vi "stateMachine_dualVStim.vi"() -> ()   [LabVIEW 2014]
uses:
  daq_channel_read_parameter.ctl
  <vilib>/Platform/TimedLoop/XDataNode/timing_clust.ctl
  <vilib>/Platform/TimedLoop/XDataNode/nitl_modes.ctl
  <vilib>/Platform/TimedLoop/XDataNode/wakeup.ctl
  <vilib>/dex/Stream Element Allocation Mode.ctl
  states_def.ctl
  UDP_Para_def.ctl
  <vilib>/DAQmx/write.llb/DAQmx Write (Digital 1D Bool NChan 1Samp 1Line).vi
  <vilib>/platform/TimedLoop/XDataNode/XDataNode.xnode
  <vilib>/Platform/TimedLoop/XDataNode/XDNodeRunTimeDep.lvlib
  <resource>/objmgr/ni.dex.rc
panel:
  out "rightcounter":i32
  out "leftcounter":i32
  out "beh type":string
  out "vs type":string
  out "Tab Control":enum32{"State Machine"}(tab)
  in  "vsFilterPeriod_uS":i32=500 format="%#1.6f"
  in  "lickThreshold_V":fxp<+/-,16,5> format="%#.4g"
  in  "vsThreshold_V":fxp<+/-,16,5> format="%#.4g"
  in  "audioThreshold_V":fxp<+/-,16,5> format="%#.4g"
  in  "audioFilterPeriod_uS":i32=50000 format="%#1.6f"
  in  "audioOffState_V":fxp<+/-,16,5> format="%#.4g"
  out "rtFIFOsize":u32=50
  out "rtFIFOtimeout":u32
  out "rtFIFOdataPool":u32=50
  out "stateMachineCycle_uS":i64=500
  out "(Actual)":i64
  in  "delay_uS":u32
  out "IP_RT":string="192.168.137.2"
  in  "port_broadcast":u16=9091
  out "IP_host":string="192.168.137.1"
  out "port_host":u16=9090
  in  "Tab Control 2":enum32{"Data Transfer"}(tab)
  out "stream counter":u32
  out "Is Connected":bool
  out "Available Elements for Writing":i32
  out "stream writer buffer size":i32=500
  in  "rewardPeriod_uS":u32
  in  "waterOn_uS":u32
  in  "timeout_uS":u32=5000000
  in  "shockOn_uS":u32
  in  "Stop state":bool
  out "Initial data received":bool
  out "Tab Control 3":enum32{"Current status"}(tab)
  in  "toneReward":bool
  out "ABORT":bool
  out "trialStart":bool
  out "trialDone":bool
  out "Busy":bool
  out "stateLatched":bool
  out "curKey":u32=1
  out "curState":u32
  out "rtFIFOdataDim":i32
  in  "actuatorOn":bool
  in  "manualWaterRight":bool
  in  "manualWaterLeft":bool
  in  "lickReward":bool
  in  "allowPunish":bool
  in  "forceLRswitch":bool
  in  "allowCorrection":bool
  in  "allowAutoWater":bool
  out "error out":errorcluster
  in  "trialKey":i32[](array[numeric])
  in  "rwdrefPeriod_uS":u32
  out "FlagWaterLeft":bool
  in  "chanellParaCluster":T1={"audioOffState_V"=0.0, "audioFilterPeriod_uS"=50000, "audioThreshold_V"=0.0, "vsThreshold_V"=0.0, "vsFilterPeriod_uS"=0, "lickThreshold_V"=0.0} {"vsFilterPeriod_uS" format="%#1.6f"; "audioFilterPeriod_uS" format="%#1.6f"}
  out "leftWaterOnFlag":bool
  out "rightWaterOnFlag":bool
  out "contNoReward":i32
  out "rewardStatus":bool
  in  "timeVS_uS":u32=2000000
  in  "timeTravel_uS":i32=400000
  out "skipRewFlag":bool
types:
  T1 = typedef "daq_channel_read_parameter.ctl" = cluster{"audioOffState_V":fxp<+/-,16,5>, "audioFilterPeriod_uS":i32, "audioThreshold_V":fxp<+/-,16,5>, "vsThreshold_V":fxp<+/-,16,5>, "vsFilterPeriod_uS":i32, "lickThreshold_V":fxp<+/-,16,5>}
  T2 = typedef "XDNodeRunTimeDep.lvlib/timing_clust.ctl" = cluster{"Expected End [f-1]":u64, "Actual End [f-1]":u64, "Finished Late? [f-1]":bool, "Expected End [i-1]":u64, "Actual End [i-1]":u64, "Finished Late? [i-1]":bool, "Expected Start [i]":u64, "Actual Start [i]":u64, "Expected Start [f]":u64, "Actual Start [f]":u64, "Source Name":string, "Structure Name":string, "Period":i64, "Deadline":i64, "Offset":i64, "Start":i64, "Priority":i32, "Timeout":i32, "Mode":T3, "Wakeup Reason":T4, "Error":errorcluster, "Source Type":string, "Secondary Source Type":string, "Global End Time":u64, "Global Start Time":u64, "Frame Duration":u64, "Iteration Duration":u64, "Assigned CPU":i32, "I/O Scan Engine Mode":u32}
  T3 = typedef "XDNodeRunTimeDep.lvlib/nitl_modes.ctl" = enum32{"No Change", "Process missed periods, maintain original phase", "Discard missed periods, maintain original phase", "Process missed periods, ignore original phase", "Discard missed periods, ignore original phase"}
  T4 = typedef "XDNodeRunTimeDep.lvlib/wakeup.ctl" = enum32{"Normal", "Aborted", "Asynchronous wakeup", "Timing source error", "Timed loop error", "Timeout"}
  T5 = typedef "states_def.ctl" = enum16{"idle", "vs before", "vs", "vs after", "delay", "tone before", "tone", "tone after", "cycle end", "reward", "reward refractory", "punish", "punish refractory", "timeout", "exit", "manualwater"}
  T6 = typedef "Stream Element Allocation Mode.ctl" = u32
  T7 = typedef "UDP_Para_def.ctl" = enum16{"no", "start", "stop", "dly", "rwp", "rwf", "wdr", "shd", "tod", "lkr", "tlr", "alp", "msh", "mwl", "mwr", "alc", "lth", "vth", "ath", "aof", "afp", "vfp"}
  T8 = cluster{"leftLick":bool, "rightLick":bool, "visualStimuli2":bool, "tone":bool, "visualStimuli1":bool}
  T9 = cluster{"leftLick":dbl, "rightLick":dbl, "visualStimuli2":dbl, "tone":dbl, "visualStimuli1":dbl}
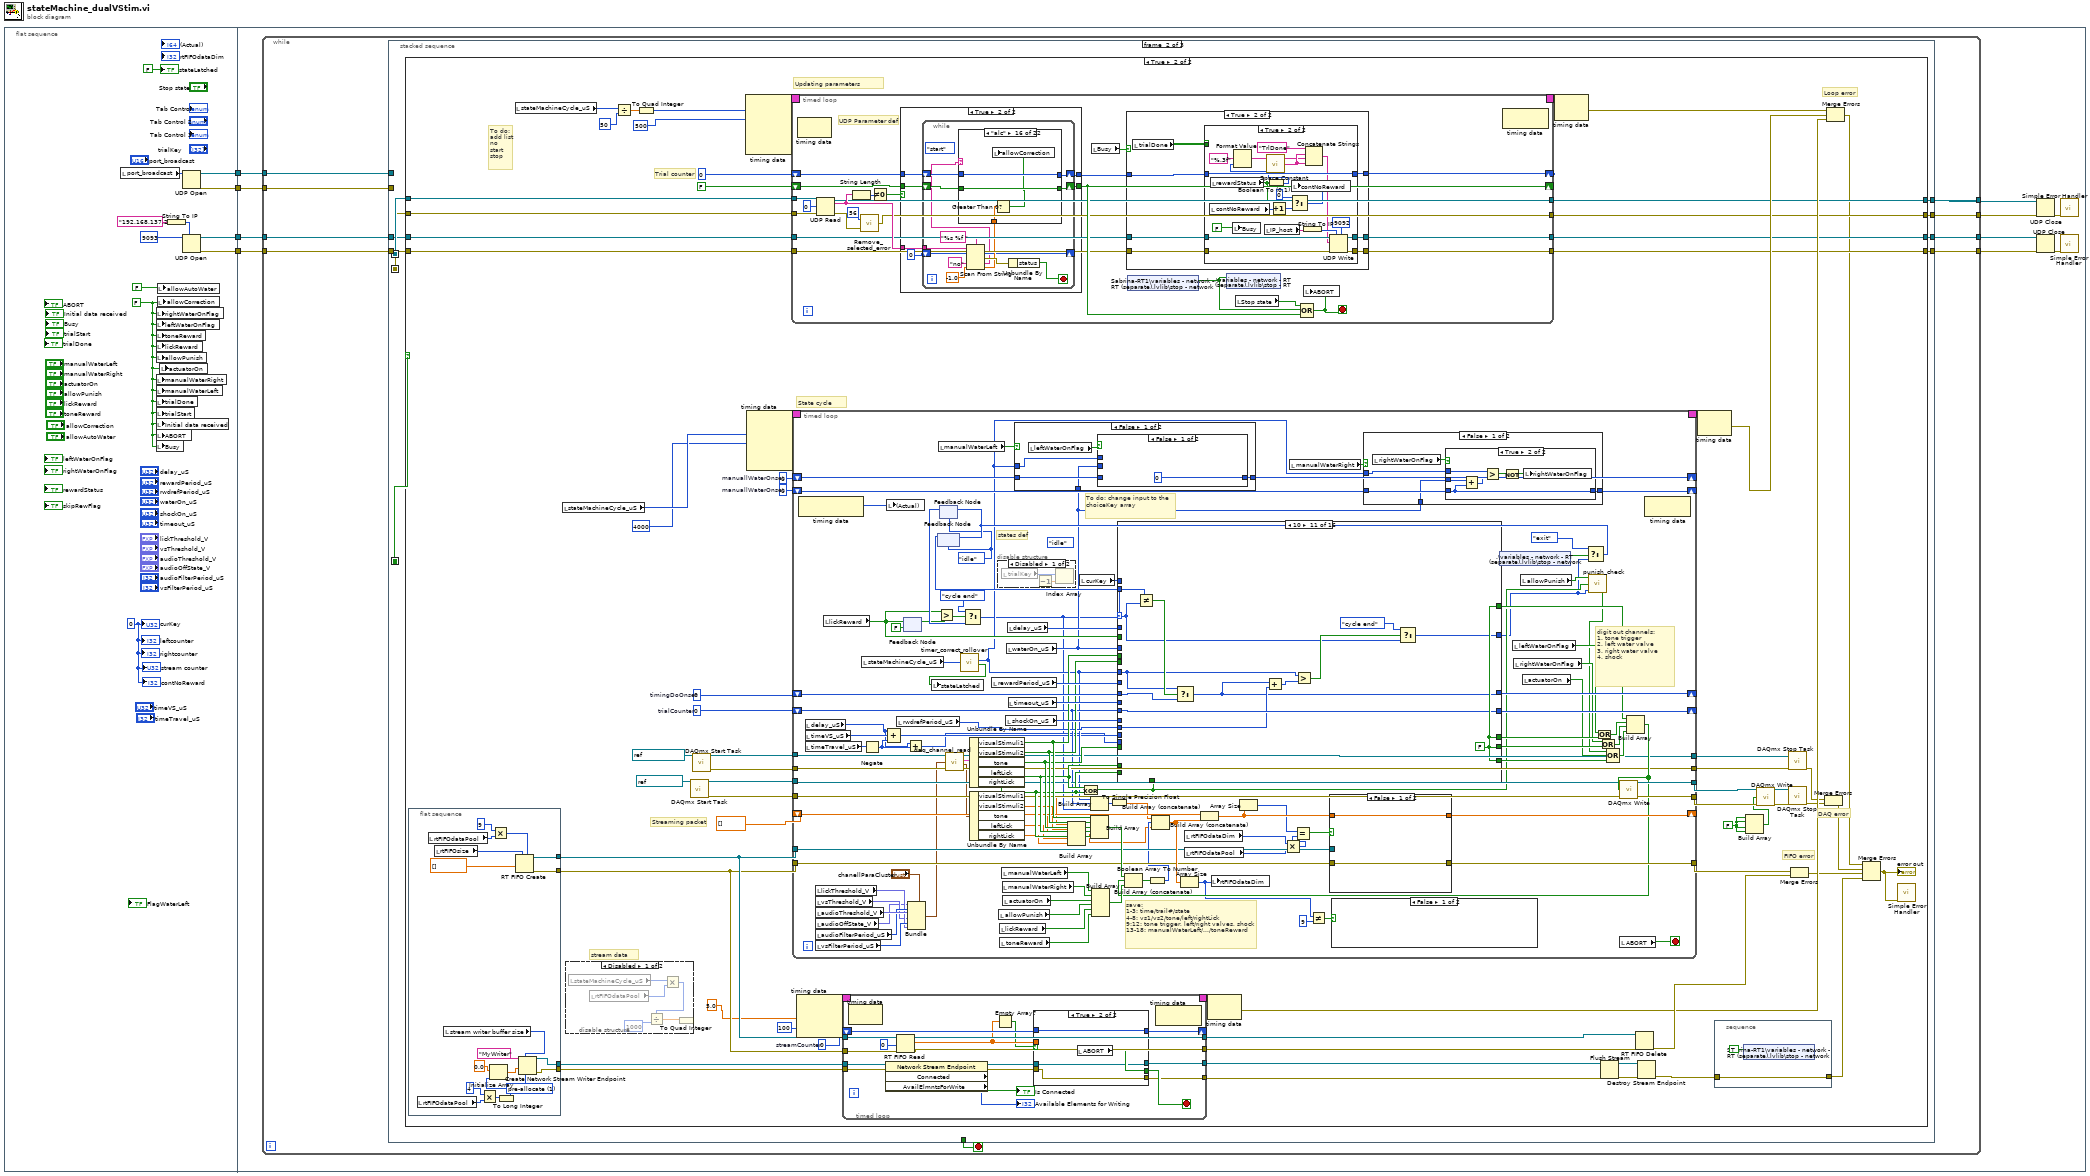
[diagram p0: block diagram]
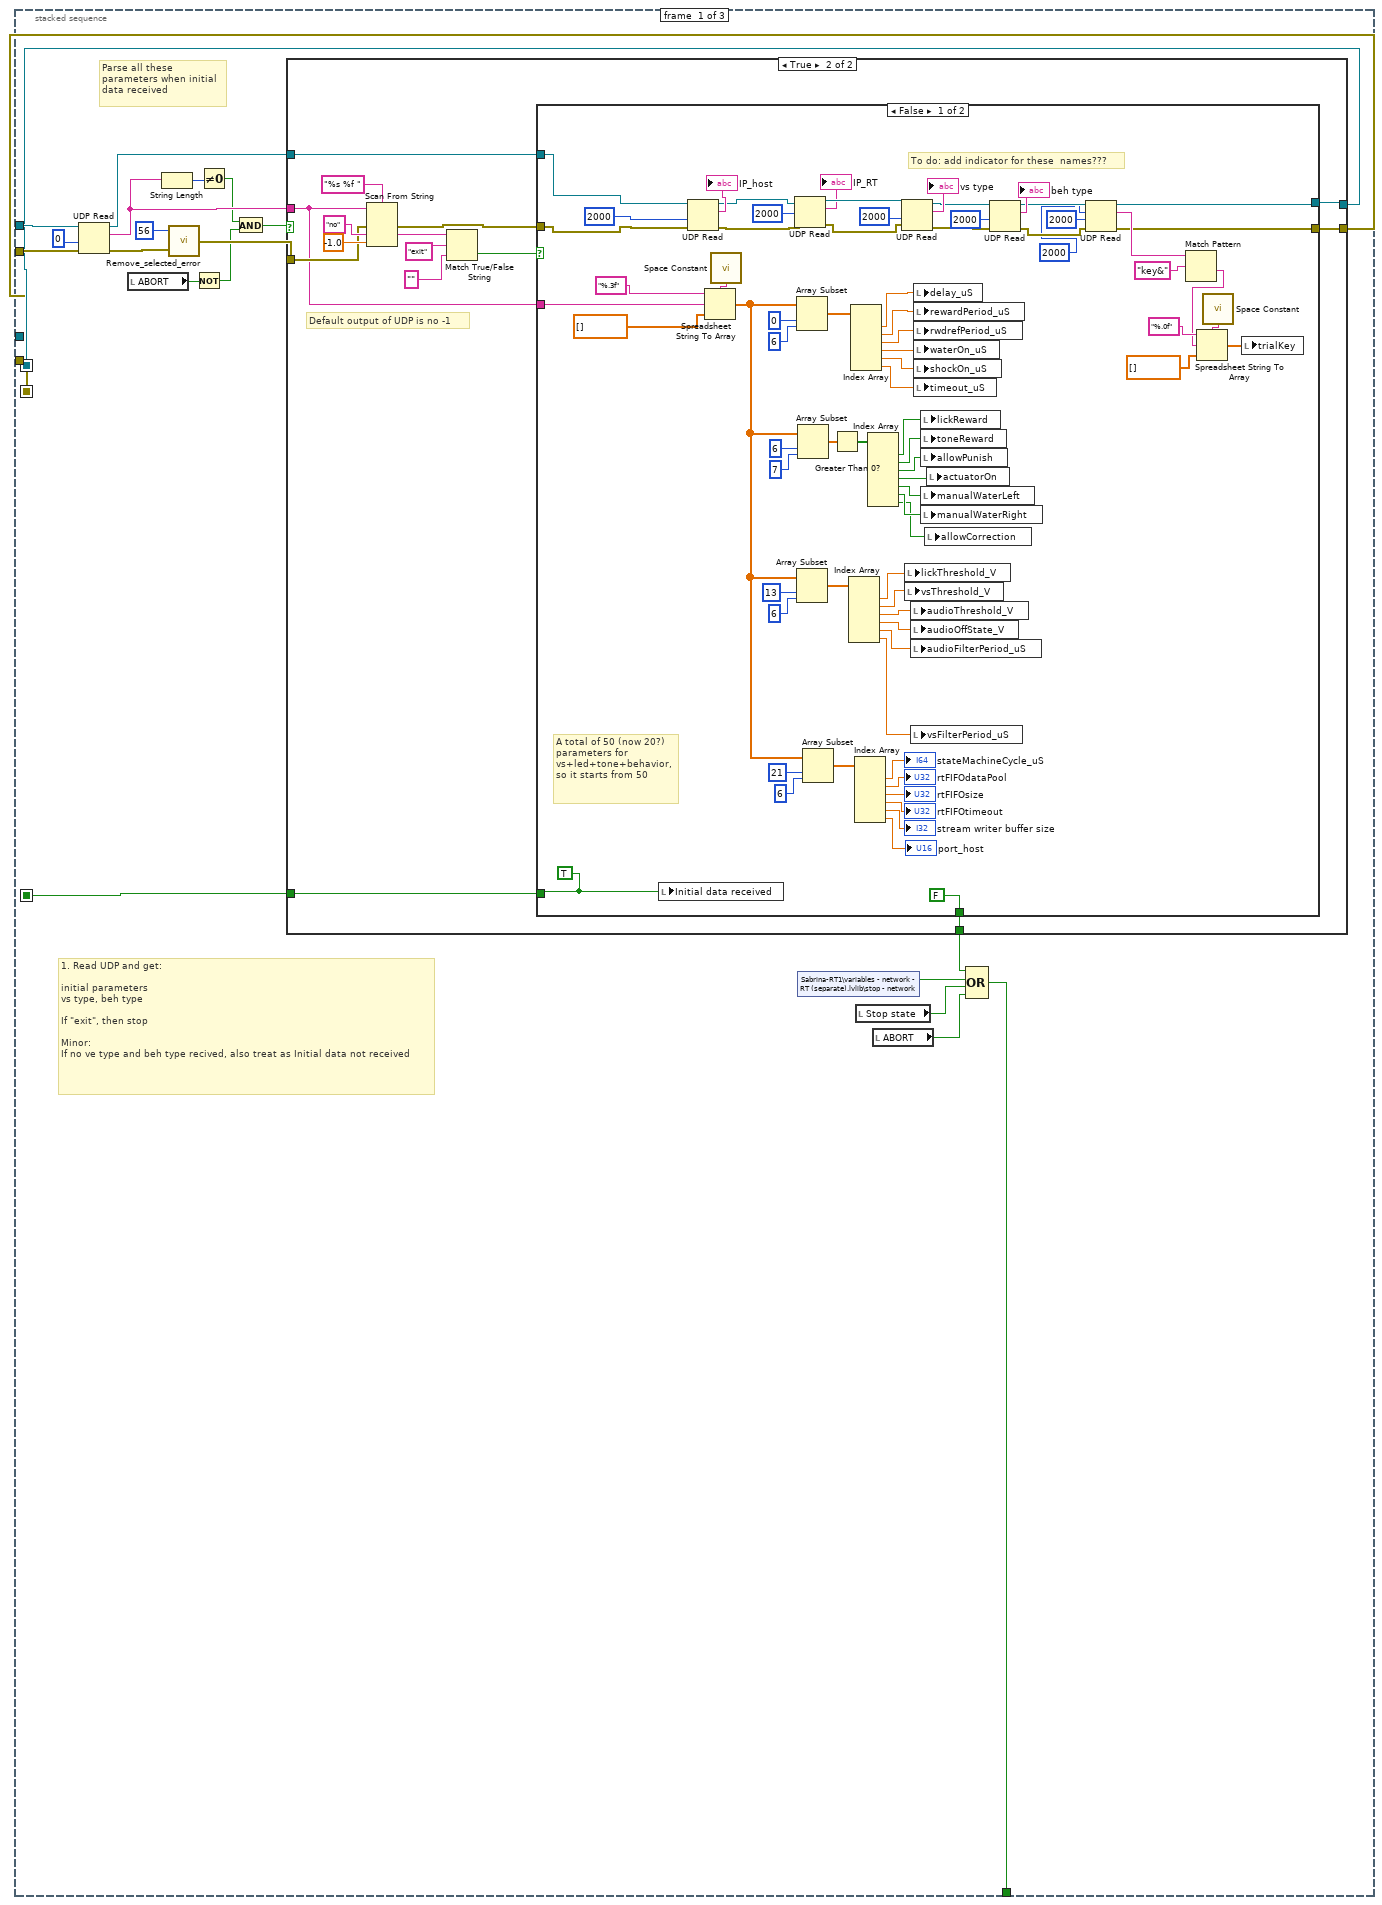
[diagram p2: hidden frame]
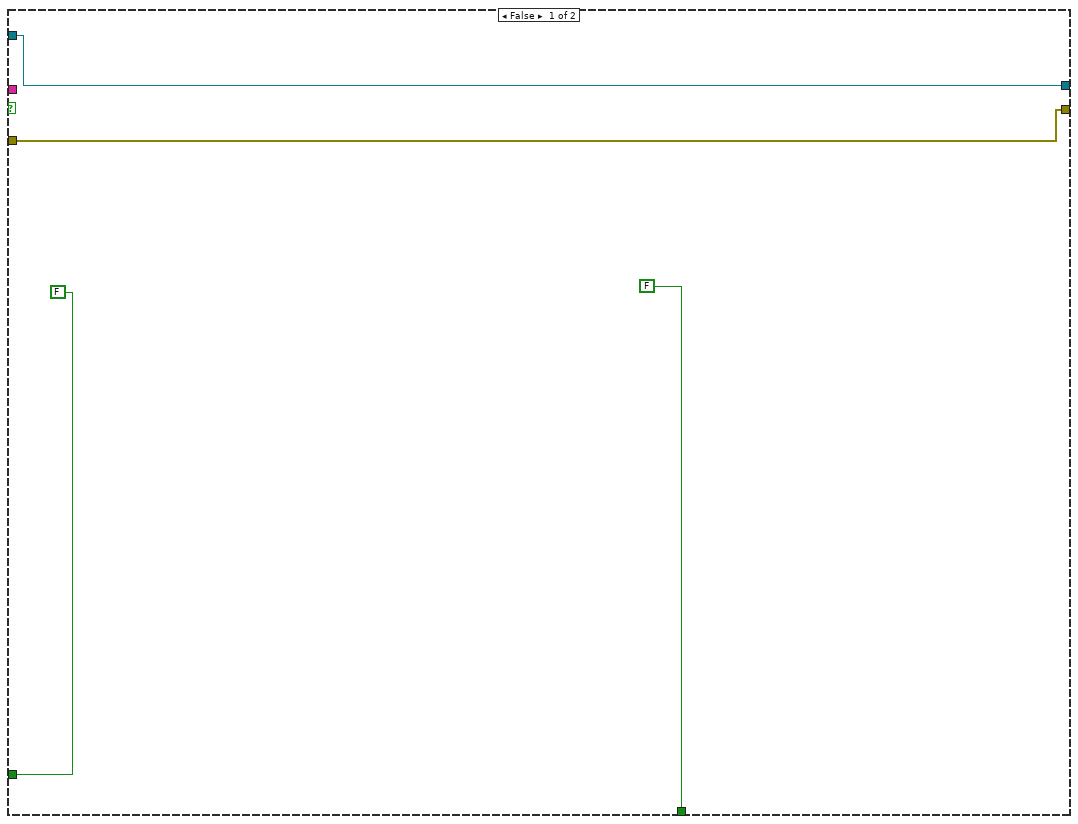
[diagram p3: hidden frame]
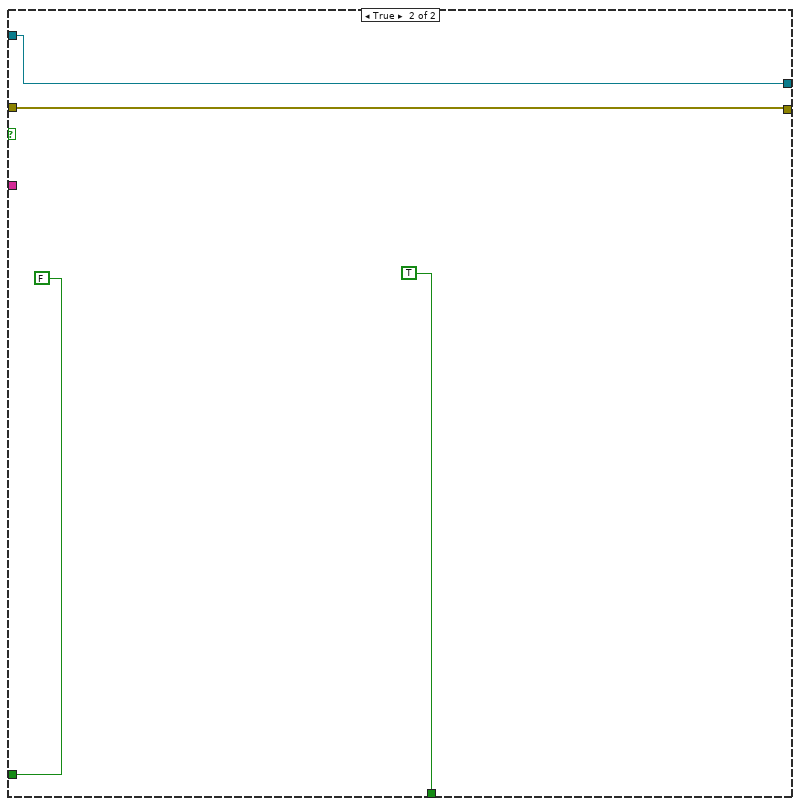
[diagram p4: hidden frame]
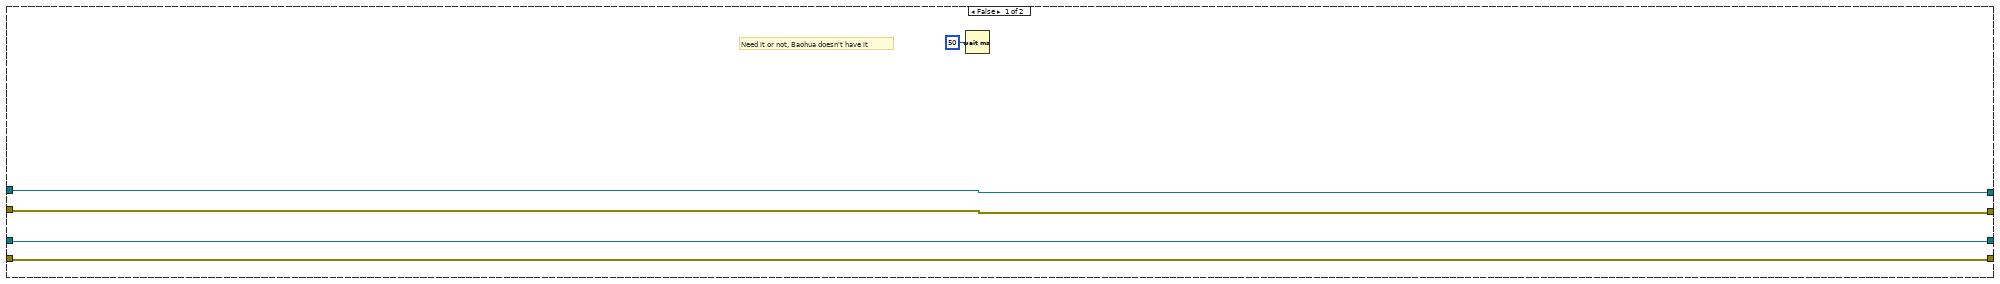
[diagram p5: hidden frame]
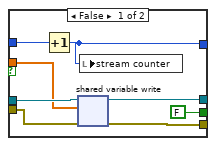
[diagram p7: hidden frame]
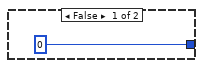
[diagram p9: hidden frame]
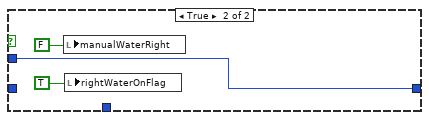
[diagram p10: hidden frame]
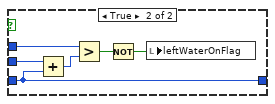
[diagram p11: hidden frame]
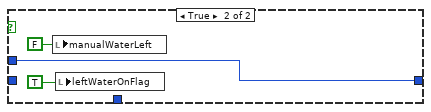
[diagram p12: hidden frame]
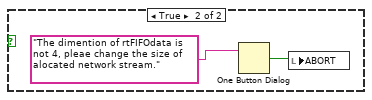
[diagram p13: hidden frame]
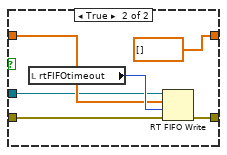
[diagram p14: hidden frame]
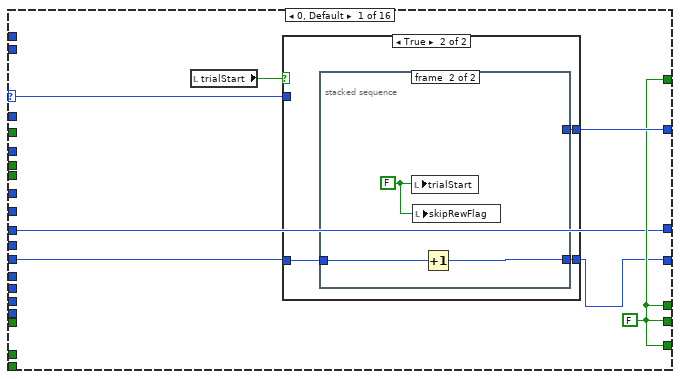
[diagram p15: hidden frame]
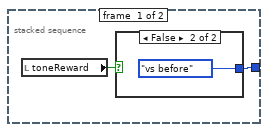
[diagram p17: hidden frame]
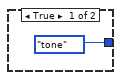
[diagram p18: hidden frame]
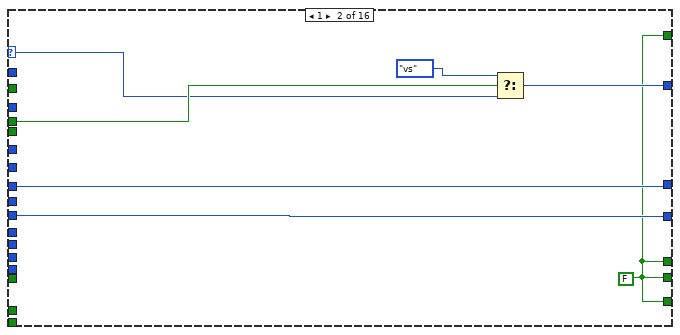
[diagram p19: hidden frame]
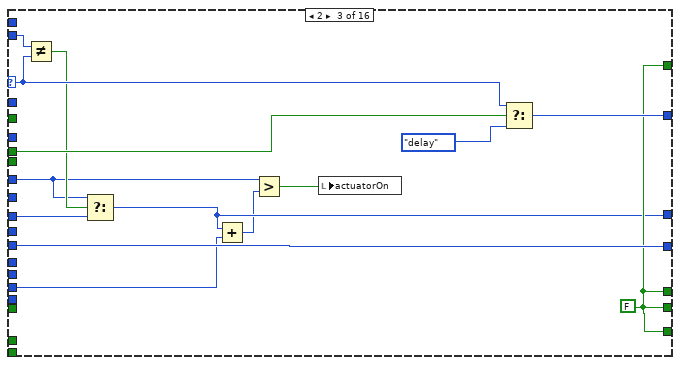
[diagram p20: hidden frame]
diagram:
  n1 = flat-sequence {
    tunnel: [w16] -> w4
    tunnel: [w15] -> w3
    tunnel: [w11] -> w2
    tunnel: [w10] -> w1
    tunnel: w4 -> [w26]
    tunnel: w3 -> [w25]
    tunnel: w2 -> [w21]
    tunnel: w1 -> [w20]
    frame #0 {
      w7 = FALSE
      w6 = 0
      n2 = local read "port_broadcast"() -> (w14:u16)
      n3 = local write "rightWaterOnFlag"(w7) -> ()
      n4 = local write "leftWaterOnFlag"(w7) -> ()
      n5 = local write "toneReward"(w7) -> ()
      n6 = local write "lickReward"(w7) -> ()
      n7 = local write "allowPunish"(w7) -> ()
      n8 = local write "manualWaterRight"(w7) -> ()
      n9 = local write "manualWaterLeft"(w7) -> ()
      n10 = local write "trialDone"(w7) -> ()
      n11 = local write "trialStart"(w7) -> ()
      n12 = local write "Initial data received"(w7) -> ()
      n13 = local write "ABORT"(w7) -> ()
      n14 = local write "Busy"(w7) -> ()
      n15 = local write "allowAutoWater"(FALSE) -> ()
      n16 = local write "allowCorrection"(w7) -> ()
      n17 = local write "actuatorOn"(w7) -> ()
      n18 = String To IP(1:"192.168.137.2") -> (0:w8:u32)
      n19 = UDP Open(7:w8, 11:u16 9093) -> (port=w11:refnum<k16>, 0:w10:errorcluster)  [unwired: 3 in, 1 out]
      n20 = UDP Open(11:w14) -> (port=w16:refnum<k16>, 0:w15:errorcluster)  [unwired: 4 in, 1 out]
      "stateLatched" <- FALSE
      "curKey" <- w6
      "leftcounter" <- w6
      "rightcounter" <- w6
      "stream counter" <- w6
      "contNoReward" <- w6
    }
    frame #1 {
      n21 = while {
        tunnel: w26 -> [w35]
        tunnel: w25 -> [w34]
        tunnel: [w32] -> w23
        tunnel: [w31] -> w22
        tunnel: w21 -> [w30]
        tunnel: w20 -> [w29]
        tunnel: [w28] -> w19
        tunnel: [w27] -> w18
        stop <- w33 stop-if-true
        n22 = stacked-sequence {
          seq-local: [w45 _ _] -> [_ w162 _]
          seq-local: [w37 _ _] -> [_ w159 _]
          seq-local: [w36 _ _] -> [_ w158 _]
          tunnel: w35 -> [w56 _ _]
          tunnel: w34 -> [w55 _ _]
          tunnel: [w46 _ _] -> w33
          tunnel: [_ w161 _] -> w32
          tunnel: [_ w160 _] -> w31
          tunnel: w30 -> [_ w157 _]
          tunnel: w29 -> [_ w154 _]
          tunnel: [_ w156 _] -> w28
          tunnel: [_ w155 _] -> w27
          frame #0 {
            # "Parse all these \nparameters when initial\ndata received"
            # "1. Read UDP and get:\n\ninitial parameters\nvs type, beh type\n\nIf \"exit\", then stop\n\nMinor:\nIf no ve type and beh type recived, also treat as Initial data not received"
            n23 = UDP Read(connection ID=w56, timeout ms (25000)=0, 8:w55) -> (data out=w53:string, error out=w43:errorcluster, 3:w54:refnum<k16>)  [unwired: 1 in, 2 out]
            n24 = local read "ABORT"() -> (w41:bool)
            n25 = String Length(string=w53) -> (length=w52:i32)
            n26 = call "Remove_selected_error.vi"("error in (no error)"=w43, "errorCode"=56 ("timeout ms (25000)")) -> ("error out"=w44:errorcluster)
            n27 = Not(x=w41) -> (.not. x?=w38:bool)
            n28 = Not Equal To 0?(x=w52) -> (x != 0?=w39:bool)
            n29 = And(x=w39, y=w38) -> (x .and. y?=w40:bool)
            n30 = case shown="True" w40 {
              tunnel: w53 -> [_ w65]
              tunnel: w54 -> [w58 w66]
              tunnel: w44 -> [w57 w73]
              tunnel: [FALSE w64] -> w50
              tunnel: [FALSE w63] -> w45
              tunnel: [w58 w62] -> w37
              tunnel: [w57 w61] -> w36
              frame False {
              }
              frame True {
                # "Default output of UDP is no -1"
                n31 = Scan From String(format string="%s %f ", input string=w65, error in=w73, default 1="no" ("default value 1"), default 2=sgl -1.0 ("default value 1")) -> (error out=w67:errorcluster, output 1=w72:string)  [unwired: 2 in, 2 out]
                n32 = Match True/False String(2:"" ("false string"), 3:"exit" ("true string"), 4:w72) -> (0:w68:bool)  [unwired: 1 out]
                n33 = case shown="False" w68 {
                  tunnel: w67 -> [w111 w151]
                  tunnel: w66 -> [w112 w150]
                  tunnel: w65 -> [w143 _]
                  tunnel: [FALSE TRUE] -> w64
                  tunnel: [w141 FALSE] -> w63
                  tunnel: [w78 w150] -> w62
                  tunnel: [w77 w151] -> w61
                  frame False {
                    w141 = TRUE
                    # "A total of 50 (now 20?) parameters for vs+led+tone+behavior, so it starts from 50"
                    # "To do: add indicator for these  names???"
                    n34 = local write "Initial data received"(w141) -> ()
                    n35 = UDP Read(connection ID=w112, timeout ms (25000)=2000, 8:w111) -> (data out=→"IP_host":string, error out=w110:errorcluster, 3:w108:refnum<k16>)  [unwired: 1 in, 2 out]
                    n36 = call <vilib>:"Space Constant.vi"() -> ("String"=w148:string)
                    n37 = Spreadsheet String To Array(delimiter (Tab)=w148, format string="%.3f", spreadsheet string=w143, array type (2D Dbl)=sgl[] []) -> (array=w119:sgl[])
                    n38 = UDP Read(connection ID=w108, timeout ms (25000)=2000, 8:w110) -> (data out=→"IP_RT":string, error out=w109:errorcluster, 3:w107:refnum<k16>)  [unwired: 1 in, 2 out]
                    n39 = Array Subset(array=w119, index=0 ("timeout ms (25000)"), length=6 ("timeout ms (25000)")) -> (w137:sgl[])
                    n40 = Array Subset(array=w119, index=13 ("timeout ms (25000)"), length=6 ("timeout ms (25000)")) -> (w133:sgl[])
                    n41 = Array Subset(array=w119, index=6 ("timeout ms (25000)"), length=7 ("timeout ms (25000)")) -> (w130:sgl[])
                    n42 = Array Subset(array=w119, index=21 ("timeout ms (25000)"), length=6 ("timeout ms (25000)")) -> (w120:sgl[])
                    n43 = Greater Than 0?(x=w130) -> (x > 0?=w129:bool[])
                    n44 = Index Array(array=w133) -> (element #1=w95:sgl, element #2=w94:sgl, element #3=w93:sgl, element #4=w92:sgl, element #5=w91:sgl, element #6=w90:sgl)  [unwired: 6 in]
                    n45 = Index Array(array=w137) -> (element #1=w101:sgl, element #2=w100:sgl, element #3=w99:sgl, element #4=w98:sgl, element #5=w97:sgl, element #6=w96:sgl)  [unwired: 6 in]
                    n46 = Index Array(array=w120) -> (element #1=→"stateMachineCycle_uS":sgl, element #2=→"rtFIFOdataPool":sgl, element #3=→"rtFIFOsize":sgl, element #4=→"rtFIFOtimeout":sgl, element #5=→"stream writer buffer size":sgl, element #6=→"port_host":sgl)  [unwired: 6 in]
                    n47 = Index Array(array=w129) -> (element #1=w128:bool, element #2=w127:bool, element #3=w126:bool, element #4=w125:bool, element #5=w124:bool, element #6=w123:bool, element #7=w76:bool)  [unwired: 7 in]
                    n48 = UDP Read(connection ID=w107, timeout ms (25000)=2000, 8:w109) -> (data out=→"vs type":string, error out=w140:errorcluster, 3:w139:refnum<k16>)  [unwired: 1 in, 2 out]
                    n49 = local write "lickThreshold_V"(w95) -> ()
                    n50 = local write "vsThreshold_V"(w94) -> ()
                    n51 = local write "audioThreshold_V"(w93) -> ()
                    n52 = local write "audioOffState_V"(w92) -> ()
                    n53 = local write "audioFilterPeriod_uS"(w91) -> ()
                    n54 = local write "vsFilterPeriod_uS"(w90) -> ()
                    n55 = local write "delay_uS"(w101) -> ()
                    n56 = local write "rewardPeriod_uS"(w100) -> ()
                    n57 = local write "rwdrefPeriod_uS"(w99) -> ()
                    n58 = local write "waterOn_uS"(w98) -> ()
                    n59 = local write "shockOn_uS"(w97) -> ()
                    n60 = local write "timeout_uS"(w96) -> ()
                    n61 = local write "lickReward"(w128) -> ()
                    n62 = local write "toneReward"(w127) -> ()
                    n63 = local write "allowPunish"(w126) -> ()
                    n64 = local write "manualWaterLeft"(w124) -> ()
                    n65 = local write "manualWaterRight"(w123) -> ()
                    n66 = local write "allowCorrection"(w76) -> ()
                    n67 = local write "actuatorOn"(w125) -> ()
                    n68 = UDP Read(connection ID=w139, timeout ms (25000)=2000, 8:w140) -> (data out=→"beh type":string, error out=w87:errorcluster, 3:w88:refnum<k16>)  [unwired: 1 in, 2 out]
                    n69 = UDP Read(connection ID=w88, max size (548)=2000 ("timeout ms (25000)"), timeout ms (25000)=2000, 8:w87) -> (data out=w82:string, error out=w77:errorcluster, 3:w78:refnum<k16>)  [unwired: 2 out]
                    n70 = Match Pattern(string=w82, regular expression="key&") -> (after substring=w80:string)  [unwired: 1 in, 3 out]
                    n71 = call <vilib>:"Space Constant.vi"() -> ("String"=w85:string)
                    n72 = Spreadsheet String To Array(delimiter (Tab)=w85, format string="%.0f", spreadsheet string=w80, array type (2D Dbl)=dbl[] []) -> (array=w83:dbl[])
                    n73 = local write "trialKey"(w83) -> ()
                  }
                  frame True {
                  }
                }
              }
            }
            n74 = shared-variable "Sabrina-RT1\\variables - network - RT (separate).lvlib\\stop - network"() -> (w49:bool)  [unwired: 1 in, 1 out]
            n75 = local read "Stop state"() -> (w48:bool)
            n76 = local read "ABORT"() -> (w47:bool)
            n77 = Compound Arithmetic op=OR(w50, w49, w48, w47) -> (w46:bool)
          }
          frame #1 {
            n78 = case shown="True" w162 {
              tunnel: w159 -> [w166 w212]
              tunnel: w158 -> [w165 w211]
              tunnel: [w166 w184] -> w161
              tunnel: [w165 w185] -> w160
              tunnel: w157 -> [w164 w189]
              tunnel: w154 -> [w163 w188]
              tunnel: [w163 w187] -> w156
              tunnel: [w164 w186] -> w155
              frame False {
                # "Need it or not, Baohua doesn't have it"
                n79 = Wait (ms)(milliseconds to wait=u32 50) -> ()  [unwired: 1 out]
              }
              frame True {
                w168 = 0  # manuallWaterOnset
                w169 = 0  # manuallWaterOnset
                w195 = FALSE
                w224 = 0  # streamCounter
                w227 = 0  # timingDoOnset
                w226 = 0  # trialCounter
                # "Streaming packet"
                # "Trial counter"
                # "Loop error"
                # "DAQ error"
                # "FIFO error"
                # "Updating parameters"
                # "State cycle"
                # "To do:\nadd list\nno\nstart\nstop"
                # "stream data"
                n80 = flat-sequence {
                  tunnel: [w254] -> w229
                  tunnel: [w253] -> w228
                  tunnel: [w252] -> w215
                  tunnel: [w251] -> w214
                  frame #0 {
                    w258 = T6 1 items=["allocate as needed", "pre-allocate"] ("element allocation mode")
                    n81 = local read "rtFIFOdataPool"() -> (w249:u32)
                    n82 = local read "rtFIFOdataPool"() -> (w246:u32)
                    n83 = local read "rtFIFOsize"() -> (w260:u32)
                    n84 = local read "stream writer buffer size"() -> (w250:i32)
                    n85 = Multiply(x=u32 4, y=w249) -> (x*y=w244:u32)
                    n86 = Multiply(x=9, y=w246) -> (x*y=w245:u32)
                    n87 = To Long Integer(number=w244) -> (32bit integer=w243:i32)
                    n88 = Initialize Array(sgl 0.0, w243) -> (w257:sgl[])
                    n89 = RT FIFO Create(1:sgl[] [], 4:w260, 6:w245) -> (8:w252:refnum<k33>, 11:w251:errorcluster)  [unwired: 5 in, 1 out]
                    n90 = Create Network Stream Writer Endpoint(6:w258, 7:w250, 9:w257, 11:"MyWriter" ("writer name")) -> (0:w254:errorcluster, 3:w253:refnum<k21>)  [unwired: 3 in]
                  }
                }
                n91 = local read "stateMachineCycle_uS"() -> (w213:i64)
                n92 = local read "stateMachineCycle_uS"() -> (w223:i64)
                n93 = disable-structure shown="Disabled" {
                  frame Disabled {
                    n94 = local read "stateMachineCycle_uS"() -> (w238:i64)
                    n95 = local read "rtFIFOdataPool"() -> (w237:u32)
                    n96 = Multiply(x=w238, y=w237) -> (x*y=w239:i64)
                    n97 = Divide(x=w239, y=i64 1000) -> (x/y=w236:dbl)
                    n98 = To Quad Integer(1:w236) -> ()  [unwired: 1 out]
                  }
                  frame Enabled {
                  }
                }
                n99 = Divide(x=w213, y=i64 50) -> (x/y=w219:dbl)
                n100 = To Quad Integer(1:w219) -> (0:w218:i64)
                n101 = call <vilib>:"DAQmx Start Task.vi"("task/channels in"=refnum<k21> "digitWrite" ("digitWrite")) -> ("task out"=w181:refnum<k21>, "error out"=w180:errorcluster)  [unwired: 13 in]
                n102 = call <vilib>:"DAQmx Start Task.vi"("task/channels in"=refnum<k21> "analogRead" ("DAQmx Task Name")) -> ("task out"=w171:refnum<k21>, "error out"=w170:errorcluster)  [unwired: 13 in]
                n103 = node-c288(w218, 500 ("Priority")) -> (w235:T2)  [unwired: 3 in]
                n104 = node-c288(w223, 4000 ("Priority")) -> (w233:T2)  [unwired: 3 in]
                n105 = timed-loop {
                  timing: w235 -> [_]
                  timing-out: [_] -> w234
                  shift-right: [w761] -> _
                  shift-left: 0 ("timeout ms (25000)") -> [w763]
                  shift-right: [w757] -> _
                  shift-left: FALSE -> [w760]
                  tunnel: [w754] -> w186
                  tunnel: [w753] -> w187
                  tunnel: w212 -> [w752]
                  tunnel: w211 -> [w751]
                  tunnel: w189 -> [w745]
                  tunnel: w188 -> [w748]
                  tunnel: [w747] -> w185
                  tunnel: [w746] -> w184
                  stop <- w759 stop-if-true
                  # "UDP Parameter def"
                  n106 = node-c288() -> ()  [unwired: 1 in, 1 out]
                  n107 = UDP Read(connection ID=w752, timeout ms (25000)=0, 8:w751) -> (data out=w764:string, error out=w750:errorcluster, 3:w746:refnum<k16>)  [unwired: 1 in, 2 out]
                  n108 = String Length(string=w764) -> (length=w766:i32)
                  n109 = call "Remove_selected_error.vi"("error in (no error)"=w750, "errorCode"=56 ("timeout ms (25000)")) -> ("error out"=w747:errorcluster)
                  n110 = Not Equal To 0?(x=w766) -> (x != 0?=w765:bool)
                  n111 = case shown="True" w765 {
                    tunnel: w764 -> [_ w808]
                    tunnel: w763 -> [w802 w807]
                    tunnel: [w802 w806] -> w762
                    tunnel: w760 -> [w801 w805]
                    tunnel: [w801 w804] -> w757
                    frame False {
                    }
                    frame True {
                      n112 = while {
                        tunnel: w808 -> [w822]
                        shift-right: [w810] -> _
                        shift-left: 0 ("timeout ms (25000)") -> [w811]
                        shift-right: [w815] -> w806
                        shift-left: w807 -> [w816]
                        shift-right: [w813] -> w804
                        shift-left: w805 -> [w814]
                        stop <- w817 stop-if-true
                        (unwired) UDP_Para_def."start"
                        n113 = Scan From String(format string="%s %f ", input string=w822, initial scan location=w811, default 1="no" ("default value 1"), default 2=-1.0 ("default value 2")) -> (offset past scan=w810:u32, error out=w818:errorcluster, output 1=w809:string, output 2=w812:dbl)  [unwired: 1 in, 1 out]
                        n114 = case shown="\"alc\"" w809 {
                          tunnel: [w824 w826 w835 w837 w842 w847 w852 w857 w862 w867 w871 w875 w879 w883 w887 w892 w895 w899 w903 w907 w911 w916] -> w815
                          tunnel: w816 -> [w824 w827 w835 w837 w842 w847 w852 w857 w862 w867 w871 w875 w879 w883 w887 w892 w895 w899 w903 w907 w911 w916]
                          tunnel: [w823 w831 w832 w836 w841 w846 w851 w856 w861 w866 w870 w874 w878 w882 w886 w891 w894 w898 w902 w906 w910 w915] -> w813
                          tunnel: w814 -> [w823 w831 w833 w836 w841 w846 w851 w856 w861 w866 w870 w874 w878 w882 w886 w891 w894 w898 w902 w906 w910 w915]
                          tunnel: w812 -> [_ w828 _ w839 w844 w849 w854 w859 w864 w869 w873 w877 w881 w885 w889 w893 w897 w901 w905 w909 w913 w918]
                          frame "no", Default {
                          }
                          frame "start" {
                            w830 = TRUE
                            n115 = Increment(x=w827) -> (x+1=w826:i32)
                            n116 = local write "rewardStatus"(FALSE) -> ()
                            n117 = local write "trialDone"(FALSE) -> ()
                            n118 = local write "Busy"(w830) -> ()
                            n119 = local write "trialStart"(w830) -> ()
                            n120 = local write "curKey"(w828) -> ()
                          }
                          frame "stop" {
                            n121 = Or(x=w833, y=TRUE) -> (x .or. y?=w832:bool)
                          }
                          frame "dly" {
                            n122 = Multiply(x=1.0, y=w839) -> (x*y=w838:dbl)
                            n123 = local write "delay_uS"(w838) -> ()
                          }
                          frame "rwp" {
                            n124 = Multiply(x=1.0, y=w844) -> (x*y=w843:dbl)
                            n125 = local write "rewardPeriod_uS"(w843) -> ()
                          }
                          frame "rwf" {
                            n126 = Multiply(x=1.0, y=w849) -> (x*y=w848:dbl)
                            n127 = local write "rwdrefPeriod_uS"(w848) -> ()
                          }
                          frame "wdr" {
                            n128 = Multiply(x=1.0, y=w854) -> (x*y=w853:dbl)
                            n129 = local write "waterOn_uS"(w853) -> ()
                          }
                          frame "shd" {
                            n130 = Multiply(x=1.0, y=w859) -> (x*y=w858:dbl)
                            n131 = local write "shockOn_uS"(w858) -> ()
                          }
                          frame "tod" {
                            n132 = Multiply(x=1.0, y=w864) -> (x*y=w863:dbl)
                            n133 = local write "timeout_uS"(w863) -> ()
                          }
                          frame "lkr" {
                            n134 = Greater Than 0?(x=w869) -> (x > 0?=w868:bool)
                            n135 = local write "lickReward"(w868) -> ()
                          }
                          frame "tlr" {
                            n136 = Greater Than 0?(x=w873) -> (x > 0?=w872:bool)
                            n137 = local write "toneReward"(w872) -> ()
                          }
                          frame "alp" {
                            n138 = Greater Than 0?(x=w877) -> (x > 0?=w876:bool)
                            n139 = local write "allowPunish"(w876) -> ()
                          }
                          frame "msh" {
                            n140 = Greater Than 0?(x=w881) -> (x > 0?=w880:bool)
                            n141 = local write "actuatorOn"(w880) -> ()
                          }
                          frame "mwl" {
                            n142 = Greater Than 0?(x=w885) -> (x > 0?=w884:bool)
                            n143 = local write "manualWaterLeft"(w884) -> ()
                          }
                          frame "mwr" {
                            n144 = Greater Than 0?(x=w889) -> (x > 0?=w888:bool)
                            n145 = local write "manualWaterRight"(w888) -> ()
                          }
                          frame "alc" {
                            n146 = Greater Than 0?(x=w893) -> (x > 0?=w890:bool)
                            n147 = local write "allowCorrection"(w890) -> ()
                          }
                          frame "lth" {
                            n148 = To Fixed-Point(number=w897) -> (fixed-point=w896:fxp<+/-,32,16>)  [unwired: 1 in]
                            n149 = local write "lickThreshold_V"(w896) -> ()
                          }
                          frame "vth" {
                            n150 = To Fixed-Point(number=w901) -> (fixed-point=w900:fxp<+/-,32,16>)  [unwired: 1 in]
                            n151 = local write "vsThreshold_V"(w900) -> ()
                          }
                          frame "ath" {
                            n152 = To Fixed-Point(number=w905) -> (fixed-point=w904:fxp<+/-,32,16>)  [unwired: 1 in]
                            n153 = local write "audioThreshold_V"(w904) -> ()
                          }
                          frame "aof" {
                            n154 = To Fixed-Point(number=w909) -> (fixed-point=w908:fxp<+/-,32,16>)  [unwired: 1 in]
                            n155 = local write "audioOffState_V"(w908) -> ()
                          }
                          frame "afp" {
                            n156 = Multiply(x=1.0, y=w913) -> (x*y=w912:dbl)
                            n157 = local write "audioFilterPeriod_uS"(w912) -> ()
                          }
                          frame "vfp" {
                            n158 = Multiply(x=1.0, y=w918) -> (x*y=w917:dbl)
                            n159 = local write "vsFilterPeriod_uS"(w917) -> ()
                          }
                        }
                        n160 = Unbundle By Name(w818) -> ("status"=w817:bool)
                      }
                    }
                  }
                  n161 = local read "Busy"() -> (w758:bool)
                  n162 = case shown="True" w758 {
                    tunnel: w762 -> [w770 w777]
                    tunnel: [w770 w771] -> w761
                    tunnel: w745 -> [w769 w776]
                    tunnel: [w769 w775] -> w754
                    tunnel: [w768 w774] -> w753
                    tunnel: w748 -> [w768 w773]
                    frame False {
                    }
                    frame True {
                      n163 = local read "trialDone"() -> (w772:bool)
                      n164 = case shown="True" w772 {
                        tunnel: w777 -> [w780 w795]
                        tunnel: [w780 w795] -> w771
                        tunnel: w776 -> [w779 w794]
                        tunnel: [w779 w793] -> w775
                        tunnel: [w778 w792] -> w774
                        tunnel: w772 -> [_ _]
                        tunnel: w773 -> [w778 w789]
                        frame False {
                        }
                        frame True {
                          n165 = local read "contNoReward"() -> (w783:i32)
                          n166 = local read "rewardStatus"() -> (w785:bool)
                          n167 = local write "Busy"(FALSE) -> ()
                          n168 = local read "IP_host"() -> (w790:string)
                          n169 = call <vilib>:"Space Constant.vi"() -> ("String"=w799:string)
                          n170 = Boolean To (0,1)(Boolean=w785) -> (0, 1=w786:i16)
                          n171 = Format Value(format string="%.3f", value (0)=w786) -> (output string=w797:string)  [unwired: 1 in]
                          n172 = Increment(x=w783) -> (x+1=w782:i32)
                          n173 = Select(t=0 ("timeout ms (25000)"), s=w785, f=w782) -> (s? t:f=w781:i32)
                          n174 = local write "contNoReward"(w781) -> ()
                          n175 = String To IP(1:w790) -> (0:w796:u32)
                          n176 = Concatenate Strings("TrlDone" ("data in"), w799, w797, w799) -> (w788:string)
                          n177 = UDP Write(address=w796, port or service name=u16 9092, connection ID=w794, data in=w788, 8:w789) -> (error out=w792:errorcluster, 3:w793:refnum<k16>)  [unwired: 1 in]
                        }
                      }
                    }
                  }
                  n178 = shared-variable "Sabrina-RT1\\variables - network - RT (separate).lvlib\\stop - network"() -> (w756:bool)  [unwired: 1 in, 1 out]
                  n179 = shared-variable ".\\variables - network - RT (separate).lvlib\\stop - RT"(w756) -> ()  [unwired: 1 in, 1 out]
                  n180 = local read "Stop state"() -> (w755:bool)
                  n181 = Compound Arithmetic op=OR(w755, w756, w757) -> (w759:bool)
                  n182 = local write "ABORT"(w759) -> ()
                  n183 = node-c288() -> ()  [unwired: 1 in, 1 out]
                }
                n184 = timed-loop {
                  timing: w233 -> [_]
                  timing-out: [_] -> w232
                  shift-right: [w392] -> _
                  shift-left: w226 -> [w330]
                  tunnel: [w403] -> w202
                  tunnel: [w402] -> w201
                  shift-right: [w400] -> _
                  shift-left: w227 -> [w401]
                  tunnel: w171 -> [w394]
                  tunnel: w170 -> [w360]
                  tunnel: [w332] -> w176
                  shift-right: [w385] -> _
                  shift-left: sgl[] [] ("array type (2D Dbl)") -> [w386]
                  tunnel: [w382] -> w192
                  tunnel: w215 -> [w359]
                  tunnel: w214 -> [w358]
                  tunnel: w181 -> [w348]
                  tunnel: w180 -> [w347]
                  tunnel: [w342] -> w177
                  shift-right: [w320] -> _
                  shift-left: w169 -> [w321]
                  shift-right: [w316] -> _
                  shift-left: w168 -> [w317]
                  stop <- w343 stop-if-true
                  w352 = states_def."idle"
                  (unwired) states_def."idle"
                  # "states def"
                  # "save: \n1-3: time/trail#/state\n4-8: vs1/vs2/tone/left/rightLick\n9:12: tone trigger, left/right valves, shock\n13-18: manualWaterLeft/.../toneReward"
                  # "digit out channels:\n1. tone trigger\n2. left water valve\n3. right water valve\n4. shock"
                  # "To do: change input to the choiceKey array"
                  n185 = node-c288() -> (w355:i64)  [unwired: 1 in]
                  n186 = local read "delay_uS"() -> (w301:u32)
                  n187 = local read "timeVS_uS"() -> (w305:u32)
                  n188 = local read "timeTravel_uS"() -> (w304:i32)
                  n189 = local read "lickThreshold_V"() -> (w336:fxp<+/-,16,5>)
                  n190 = local read "vsThreshold_V"() -> (w335:fxp<+/-,16,5>)
                  n191 = local read "audioThreshold_V"() -> (w341:fxp<+/-,16,5>)
                  n192 = local read "audioOffState_V"() -> (w334:fxp<+/-,16,5>)
                  n193 = local read "audioFilterPeriod_uS"() -> (w337:i32)
                  n194 = local read "vsFilterPeriod_uS"() -> (w338:i32)
                  n195 = local read "lickReward"() -> (w361:bool)
                  n196 = local read "stateMachineCycle_uS"() -> (w356:i64)
                  n197 = Negate(x=w304) -> (-x=w302:i32)
                  n198 = local write "(Actual)"(w355) -> ()
                  n199 = Compound Arithmetic op=ADD(w301, w305, w302) -> (w303:u32)
                  n200 = local read "rwdrefPeriod_uS"() -> (w349:u32)
                  n201 = feedback #1(FALSE ("lick-reward")) -> (w406:bool)
                  n202 = feedback-in #1(w361) -> ()
                  n203 = Add(x=w301, y=w302) -> (x+y=w300:u32)
                  n204 = Bundle(cluster="chanellParaCluster", "audioOffState_V"=w334, "audioFilterPeriod_uS"=w337, "audioThreshold_V"=w341, "vsThreshold_V"=w335, "vsFilterPeriod_uS"=w338, "lickThreshold_V"=w336) -> (w340:T1)
                  n205 = feedback #2(w352) -> (w404:u32)
                  n206 = Greater?(x=w361, y=w406) -> (0:w407:bool)
                  n207 = local read "manualWaterLeft"() -> (w322:bool)
                  n208 = feedback #3(w352) -> (w408:u32)
                  n209 = call "daq_channel_read.vi"("DAQmxTaskIn"=w394, "chanellParaCluster"=w340, "error in (no error)"=w360) -> ("DAQmxTaskOut"=w342:refnum<k21>, "channelOutCluster"=w333:T8, "channelOutCluster_rawData"=w331:T9, "error out"=w332:errorcluster)
                  n210 = call "timer_correct_rollover.vi"("Loop Rate(uSec)"=w356) -> ("Late? (Latched)"=w395:bool, "Tick Count(uSec)"=w315:u64)  [unwired: 8 in, 1 out]
                  n211 = local write "stateLatched"(w395) -> ()
                  n212 = Select(t=states_def."cycle end", s=w407, f=w408) -> (s? t:f=w299:u32)
                  n213 = Unbundle By Name(w333) -> ("visualStimuli1"=w391:bool, "visualStimuli2"=w390:bool, "tone"=w389:bool, "leftLick"=w388:bool, "rightLick"=w387:bool)
                  n214 = Unbundle By Name(w331) -> ("visualStimuli1"=w324:dbl, "visualStimuli2"=w329:dbl, "tone"=w328:dbl, "leftLick"=w327:dbl, "rightLick"=w326:dbl)
                  n215 = local read "rewardPeriod_uS"() -> (w398:u32)
                  n216 = disable-structure shown="Disabled" {
                    frame Disabled {
                      n217 = local read "trialKey"() -> (w411:i32[])
                      n218 = Decrement() -> (x-1=w410:dbl)  [unwired: 1 in]
                      n219 = Index Array(array=w411, index=w410) -> ()  [unwired: 1 out]
                    }
                    frame Enabled {
                    }
                  }
                  n220 = local read "allowPunish"() -> (w370:bool)
                  n221 = local read "lickReward"() -> (w371:bool)
                  n222 = local read "toneReward"() -> (w350:bool)
                  n223 = local read "manualWaterLeft"() -> (w368:bool)
                  n224 = local read "manualWaterRight"() -> (w367:bool)
                  n225 = local read "actuatorOn"() -> (w369:bool)
                  n226 = local read "shockOn_uS"() -> (w393:u32)
                  n227 = local read "waterOn_uS"() -> (w314:u32)
                  n228 = local read "delay_uS"() -> (w351:u32)
                  n229 = local read "timeout_uS"() -> (w397:u32)
                  n230 = case shown="False" w322 {
                    tunnel: w321 -> [w430 _]
                    tunnel: [w429 w441] -> w320
                    tunnel: w315 -> [w428 w441]
                    tunnel: w314 -> [w427 _]
                    frame False {
                      n231 = local read "leftWaterOnFlag"() -> (w431:bool)
                      n232 = case shown="False" w431 {
                        tunnel: w430 -> [_ w436]
                        tunnel: [0 w436] -> w429
                        tunnel: w428 -> [_ w438]
                        tunnel: w427 -> [_ w437]
                        frame False {
                        }
                        frame True {
                          n233 = Add(x=w437, y=w436) -> (x+y=w435:u64)
                          n234 = Greater?(x=w438, y=w435) -> (0:w434:bool)
                          n235 = Not(x=w434) -> (.not. x?=w433:bool)
                          n236 = local write "leftWaterOnFlag"(w433) -> ()
                        }
                      }
                    }
                    frame True {
                      n237 = local write "manualWaterLeft"(FALSE) -> ()
                      n238 = local write "leftWaterOnFlag"(TRUE) -> ()
                    }
                  }
                  n239 = Build Array(w324, w329, w328, w327, w326) -> (w323:dbl[])
                  n240 = local read "curKey"() -> (w312:u32)
                  n241 = Exclusive Or(1:w387, 2:w388) -> (0:w308:bool)
                  n242 = Build Array(w315, w330, w299) -> (w365:u64[])
                  n243 = Build Array(w391, w390, w389, w388, w387) -> (w375:bool[])
                  n244 = Build Array(w368, w367, w369, w370, w371, w350) -> (w374:bool[])
                  n245 = To Single Precision Float(number=w365) -> (single precision float=w366:sgl[])
                  n246 = case shown="10" w299 {
                    selector: w299 -> [w455 w475 w485 w498 w515 w531 w544 w553 w632 w652 w686 w694 w708 w720 w726 _]
                    tunnel: w391 -> [_ w477 w491 w497 _ _ _ _ _ _ _ _ _ _ _ _]
                    tunnel: w404 -> [_ _ w486 _ w516 _ _ _ _ w669 _ w700 _ w721 _ _]
                    tunnel: w315 -> [_ _ w480 _ w501 w526 w540 w568 w635 w667 w683 w695 _ w718 _ _]
                    tunnel: [w458 w476 w490 w496 w520 w525 w545 w567 w639 w665 w687 w698 w708 w719 w726 states_def."tone after"] -> w307
                    tunnel: w390 -> [_ _ _ _ _ _ _ _ _ _ _ _ _ _ _ _]
                    tunnel: [w456 w471 w487 w492 w513 w524 w542 w559 w636 w657 w691 w692 w707 w712 w725 w729] -> w380
                    tunnel: w361 -> [_ _ _ _ _ _ _ w557 w640 w654 _ _ _ _ _ _]
                    tunnel: w330 -> [w452 w473 w489 w494 w519 w527 w543 w562 w638 w661 w684 w704 w709 w714 w728 w730]
                    tunnel: w389 -> [_ _ _ _ _ w529 _ _ _ _ _ _ _ _ _ _]
                    tunnel: w401 -> [w454 w474 w484 w495 w512 w530 w539 w563 w634 w659 w689 w703 w710 w717 w727 w731]
                    tunnel: [w454 w474 w481 w495 w502 w528 w541 w563 w633 w658 w680 w696 w710 w715 w727 w731] -> w400
                    tunnel: w388 -> [_ _ _ _ _ _ _ w565 _ _ _ _ _ _ _ _]
                    tunnel: w387 -> [_ _ _ _ _ _ _ w564 _ _ _ _ _ _ _ _]
                    tunnel: [w456 w471 w487 w492 w513 w523 w542 w559 w636 w663 w691 w692 w707 w712 w725 w729] -> w379
                    tunnel: [w456 w471 w487 w492 w513 w523 w542 w559 w636 w662 w691 w692 w707 w712 w725 w729] -> w377
                    tunnel: [w453 w473 w489 w494 w519 w527 w543 w562 w637 w661 w684 w704 w709 w714 w728 w730] -> w392
                    tunnel: w308 -> [_ _ _ _ w504 _ _ w561 _ _ _ _ _ _ _ _]
                    tunnel: w398 -> [_ _ _ _ _ _ _ w560 _ _ _ _ _ _ _ _]
                    tunnel: w314 -> [_ _ _ _ _ _ _ _ _ w660 _ _ _ _ _ _]
                    tunnel: w397 -> [_ _ _ _ _ _ _ _ _ _ _ _ _ w716 _ _]
                    tunnel: [w456 w471 w487 w492 w513 w523 w542 w559 w636 w657 w691 TRUE w707 w712 w725 w729] -> w311
                    tunnel: w393 -> [_ _ _ _ _ _ _ _ _ _ _ w693 _ _ _ _]
                    tunnel: w351 -> [_ _ _ _ w517 _ _ _ _ _ _ _ _ _ _ _]
                    tunnel: w349 -> [_ _ _ _ _ _ _ _ _ _ w681 _ _ _ _ _]
                    tunnel: w312 -> [_ _ _ _ _ _ _ w554 _ w651 _ _ _ _ _ w733]
                    tunnel: w303 -> [_ _ w482 _ _ _ _ _ _ _ _ _ _ _ _ _]
                    tunnel: w300 -> [_ _ _ _ w503 _ _ _ _ _ _ _ _ _ _ _]
                    frame 0, Default {
                      w456 = FALSE
                      n247 = local read "trialStart"() -> (w457:bool)
                      n248 = case shown="True" w457 {
                        tunnel: [w460 w463] -> w458
                        tunnel: w455 -> [w460 _]
                        tunnel: w452 -> [w459 w462]
                        tunnel: [w459 w461] -> w453
                        frame False {
                        }
                        frame True {
                          n249 = stacked-sequence {
                            tunnel: [w464 _] -> w463
                            tunnel: w462 -> [_ w470]
                            tunnel: [_ w469] -> w461
                            frame #0 {
                              n250 = local read "toneReward"() -> (w465:bool)
                              n251 = case shown="False" w465 {
                                tunnel: [states_def."tone" states_def."vs before"] -> w464
                                frame True {
                                }
                                frame False {
                                }
                              }
                            }
                            frame #1 {
                              w468 = FALSE
                              n252 = local write "trialStart"(w468) -> ()
                              n253 = local write "skipRewFlag"(w468) -> ()
                              n254 = Increment(x=w470) -> (x+1=w469:i32)
                            }
                          }
                        }
                      }
                    }
                    frame 1 {
                      w471 = FALSE
                      n255 = Select(t=states_def."vs", s=w477, f=w475) -> (s? t:f=w476:u32)
                    }
                    frame 2 {
                      w487 = FALSE
                      n256 = Not Equal?(x=w486, y=w485) -> (x != y?=w483:bool)
                      n257 = Select(t=w480, s=w483, f=w484) -> (s? t:f=w481:u64)
                      n258 = Add(x=w481, y=w482) -> (x+y=w479:u64)
                      n259 = Greater?(x=w480, y=w479) -> (0:w478:bool)
                      n260 = local write "actuatorOn"(w478) -> ()
                      n261 = Select(t=w485, s=w491, f=states_def."delay") -> (s? t:f=w490:u32)
                    }
                    frame 3 {
                      w492 = FALSE
                      n262 = Select(t=w498, s=w497, f=states_def."delay") -> (s? t:f=w496:u32)
                    }
                    frame 4 {
                      w513 = FALSE
                      n263 = local read "allowPunish"() -> (w505:bool)
                      n264 = Not Equal?(x=w516, y=w515) -> (x != y?=w514:bool)
                      n265 = Select(t=w501, s=w514, f=w512) -> (s? t:f=w502:u64)
                      n266 = And(x=w505, y=w504) -> (x .and. y?=w506:bool)
                      n267 = case shown="True" w506 {
                        selector: w506 -> [_ w522]
                        frame False {
                        }
                        frame True {
                          n268 = local write "skipRewFlag"(w522) -> ()
                        }
                      }
                      n269 = Add(x=w517, y=w502) -> (x+y=w518:u64)
                      n270 = local read "skipRewFlag"() -> (w510:bool)
                      n271 = Less?(x=w518, y=w501) -> (x < y?=w511:bool)
                      n272 = Add(x=w502, y=w503) -> (x+y=w500:u64)
                      n273 = Select(t=states_def."timeout", s=w510, f=states_def."tone after") -> (s? t:f=w508:T5)
                      n274 = Greater?(x=w501, y=w500) -> (0:w499:bool)
                      n275 = case shown="True" w499 {
                        frame False {
                        }
                        frame True {
                          n276 = local write "actuatorOn"(TRUE) -> ()
                        }
                      }
                      n277 = Select(t=w508, s=w511, f=w515) -> (s? t:f=w520:u32)
                    }
                    frame 5 {
                      w523 = FALSE
                      n278 = case shown="True" w529 {
                        tunnel: [w534 states_def."tone after"] -> w525
                        tunnel: w531 -> [w534 _]
                        tunnel: w530 -> [w533 _]
                        tunnel: [w533 w537] -> w528
                        tunnel: w526 -> [_ w537]
                        tunnel: [TRUE FALSE] -> w524
                        frame False {
                        }
                        frame True {
                        }
                      }
                    }
                    frame 6 {
                      w542 = FALSE
                      n279 = local read "Busy"() -> (w538:bool)
                      n280 = case shown="True" w538 {
                        tunnel: [w547 states_def."tone after"] -> w545
                        tunnel: w544 -> [w547 _]
                        tunnel: w540 -> [_ w548]
                        tunnel: [w546 w548] -> w541
                        tunnel: w539 -> [w546 _]
                        frame False {
                        }
                        frame True {
                        }
                      }
                    }
                    frame 7 {
                      w559 = FALSE
                      n281 = local read "toneReward"() -> (w556:bool)
                      n282 = local read "allowAutoWater"() -> (w552:bool)
                      n283 = Or(x=w556, y=w557) -> (x .or. y?=w555:bool)
                      n284 = case shown="True" w561 {
                        tunnel: w565 -> [_ w593]
                        tunnel: w564 -> [_ w592]
                        tunnel: w555 -> [_ w591]
                        tunnel: w554 -> [_ w590]
                        tunnel: [w582 w588] -> w551
                        tunnel: w553 -> [w582 w586]
                        frame False {
                        }
                        frame True {
                          n285 = case shown="True" w591 {
                            tunnel: [w609 w623] -> w583
                            tunnel: w593 -> [w606 w622]
                            tunnel: w592 -> [w610 w621]
                            tunnel: w590 -> [_ w620]
                            frame True {
                              n286 = Not(x=w606) -> (.not. x?=w611:bool)
                              n287 = Not(x=w610) -> (.not. x?=w607:bool)
                              n288 = local read "rightcounter"() -> (w603:i32)
                              n289 = local read "leftcounter"() -> (w604:i32)
                              n290 = Select(t=3, s="forceLRswitch", f=inf) -> (s? t:f=w594:dbl)
                              n291 = Select(t=3, s="forceLRswitch", f=inf) -> (s? t:f=w600:dbl)
                              n292 = Less?(x=w603, y=w594) -> (x < y?=w602:bool)
                              n293 = Compound Arithmetic op=AND(w611, w610, w602) -> (w608:bool)
                              n294 = Less?(x=w604, y=w600) -> (x < y?=w605:bool)
                              n295 = Compound Arithmetic op=AND(w605, w606, w607) -> (w601:bool)
                              n296 = case shown="True" w601 {
                                frame False {
                                }
                                frame True {
                                n297 = local read "leftcounter"() -> (w617:i32)
                                n298 = local write "FlagWaterLeft"(TRUE) -> ()
                                n299 = Increment(x=w617) -> (x+1=w618:i32)
                                n300 = local write "leftcounter"(w618) -> ()
                                n301 = local write "rightcounter"(0) -> ()
                                }
                              }
                              n302 = case shown="True" w608 {
                                frame False {
                                }
                                frame True {
                                n303 = local read "rightcounter"() -> (w613:i32)
                                n304 = local write "FlagWaterLeft"(FALSE) -> ()
                                n305 = Increment(x=w613) -> (x+1=w612:i32)
                                n306 = local write "rightcounter"(w612) -> ()
                                n307 = local write "leftcounter"(0) -> ()
                                }
                              }
                              n308 = Exclusive Or(1:w608, 2:w601) -> (0:w609:bool)
                            }
                            frame False {
                              # "Consider add another state for automaticaly give water \nwhen animal did not get water for consecutively 10 trials?"
                              n309 = case shown="2" w620 {
                                tunnel: [w626 w628] -> w623
                                tunnel: w622 -> [w625 w631]
                                tunnel: w621 -> [w624 w629]
                                frame 1, Default {
                                # "left"
                                n310 = Not(x=w624) -> (.not. x?=w627:bool)
                                n311 = And(x=w625, y=w627) -> (x .and. y?=w626:bool)
                                }
                                frame 2 {
                                # "right"
                                n312 = Not(x=w631) -> (.not. x?=w630:bool)
                                n313 = And(x=w630, y=w629) -> (x .and. y?=w628:bool)
                                }
                              }
                            }
                          }
                          n314 = local read "allowCorrection"() -> (w585:bool)
                          n315 = Select(t=w586, s=w585, f=states_def."timeout") -> (s? t:f=w584:u32)
                          n316 = Select(t=states_def."reward", s=w583, f=w584) -> (s? t:f=w588:u32)
                        }
                      }
                      n317 = case shown="True" w552 {
                        tunnel: w551 -> [w570 w580]
                        tunnel: [w570 w579] -> w550
                        frame False {
                        }
                        frame True {
                          w573 = 10 ("Priority")
                          n318 = local read "contNoReward"() -> (w577:i32)
                          n319 = Random Number (0-1)() -> (number: 0 to 1=w574:dbl)
                          n320 = Multiply(x=w574, y=w573) -> (x*y=w572:dbl)
                          n321 = Add(x=w572, y=w573) -> (x+y=w571:dbl)
                          n322 = Greater Or Equal?(x=w577, y=w571) -> (x >= y?=w576:bool)
                          n323 = Select(t=0 ("Priority"), s=w576, f=w577) -> (s? t:f=w575:i32)
                          n324 = Select(t=states_def."manualwater", s=w576, f=w580) -> (s? t:f=w579:u32)
                          n325 = local write "contNoReward"(w575) -> ()
                        }
                      }
                      n326 = Add(x=w560, y=w563) -> (x+y=w569:u64)
                      n327 = Greater?(x=w568, y=w569) -> (0:w566:bool)
                      n328 = Select(t=states_def."cycle end", s=w566, f=w550) -> (s? t:f=w567:u32)
                    }
                    frame 8 {
                      w636 = FALSE
                      # "inform host computer to start \nanother trial"
                      n329 = case shown="False" w640 {
                        tunnel: [w642 w648] -> w637
                        tunnel: [states_def."idle" states_def."tone after"] -> w639
                        tunnel: w638 -> [w642 w648]
                        tunnel: [w643 w646] -> w633
                        tunnel: w635 -> [w643 w646]
                        tunnel: w634 -> [_ _]
                        tunnel: w632 -> [_ _]
                        frame False {
                          n330 = local write "actuatorOn"(FALSE) -> ()
                          n331 = local write "trialDone"(TRUE) -> ()
                        }
                        frame True {
                        }
                      }
                    }
                    frame 9 {
                      w657 = FALSE
                      w649 = states_def."reward refractory"
                      n332 = Not Equal?(x=w669, y=w652) -> (x != y?=w664:bool)
                      n333 = local read "toneReward"() -> (w655:bool)
                      n334 = Select(t=w667, s=w664, f=w659) -> (s? t:f=w658:u64)
                      n335 = Or(x=w654, y=w655) -> (x .or. y?=w656:bool)
                      n336 = case shown="False" w656 {
                        tunnel: [w671 w674] -> w663
                        tunnel: [w670 w673] -> w662
                        tunnel: w651 -> [_ w672]
                        frame True {
                          n337 = local read "FlagWaterLeft"() -> (w671:bool)
                          n338 = Not(x=w671) -> (.not. x?=w670:bool)
                        }
                        frame False {
                          n339 = case shown="0, Default" w672 {
                            tunnel: [w675 w677 w678] -> w674
                            tunnel: [w675 w676 w679] -> w673
                            frame 0, Default {
                              w675 = FALSE
                            }
                            frame 1 {
                              w677 = TRUE
                              n340 = Not(x=w677) -> (.not. x?=w676:bool)
                            }
                            frame 2 {
                              w679 = TRUE
                              n341 = Not(x=w679) -> (.not. x?=w678:bool)
                            }
                          }
                        }
                      }
                      n342 = Add(x=w660, y=w658) -> (x+y=w668:u64)
                      n343 = Less?(x=w668, y=w667) -> (x < y?=w666:bool)
                      n344 = Select(t=w649, s=w654, f=states_def."cycle end") -> ()  [unwired: 1 out]
                      n345 = local write "rewardStatus"(TRUE) -> ()
                      n346 = Select(t=w649, s=w666, f=w652) -> (s? t:f=w665:u32)
                    }
                    frame 10 {
                      w691 = FALSE
                      n347 = Not Equal?(x=w686, y=w686) -> (x != y?=w690:bool)
                      n348 = Select(t=w683, s=w690, f=w689) -> (s? t:f=w680:u64)
                      n349 = Add(x=w680, y=w681) -> (x+y=w682:u64)
                      n350 = Greater?(x=w683, y=w682) -> (0:w688:bool)
                      n351 = Select(t=states_def."cycle end", s=w688, f=w686) -> (s? t:f=w687:u32)
                    }
                    frame 11 {
                      w692 = FALSE
                      n352 = Not Equal?(x=w700, y=w694) -> (x != y?=w702:bool)
                      n353 = case shown="True" w702 {
                        tunnel: w694 -> [_ w706]
                        frame False {
                        }
                        frame True {
                          "curState" <- w706
                        }
                      }
                      n354 = Select(t=w695, s=w702, f=w703) -> (s? t:f=w696:u64)
                      n355 = Add(x=w696, y=w693) -> (x+y=w697:u64)
                      n356 = Less?(x=w695, y=w697) -> (x < y?=w701:bool)
                      n357 = local read "curState"() -> (w699:u32)
                      n358 = Select(t=w694, s=w701, f=w699) -> (s? t:f=w698:u32)
                    }
                    frame 12 {
                      w707 = FALSE
                      # "To do"
                    }
                    frame 13 {
                      w712 = FALSE
                      # "To do: change the state when timeout finished?????"
                      n359 = Not Equal?(x=w721, y=w720) -> (x != y?=w724:bool)
                      n360 = Select(t=w718, s=w724, f=w717) -> (s? t:f=w715:u64)
                      n361 = local write "actuatorOn"(FALSE) -> ()
                      n362 = Add(x=w715, y=w716) -> (x+y=w723:u64)
                      n363 = Greater?(x=w718, y=w723) -> (0:w722:bool)
                      n364 = Select(t=states_def."cycle end", s=w722, f=w720) -> (s? t:f=w719:u32)
                    }
                    frame 14 {
                      w725 = FALSE
                    }
                    frame 15 {
                      w729 = FALSE
                      n365 = case shown="1" w733 {
                        frame 0, Default {
                        }
                        frame 1 {
                          n366 = local write "manualWaterLeft"(TRUE) -> ()
                        }
                        frame 2 {
                          n367 = local write "manualWaterRight"(TRUE) -> ()
                        }
                      }
                    }
                  }
                  n368 = local read "rtFIFOdataPool"() -> (w357:u32)
                  n369 = local read "rtFIFOdataDim"() -> (w362:i32)
                  n370 = Multiply(x=w362, y=w357) -> (x*y=w363:u32)
                  n371 = local read "manualWaterRight"() -> (w318:bool)
                  n372 = case shown="False" w318 {
                    tunnel: [w415 w424] -> w316
                    tunnel: w317 -> [w416 _]
                    tunnel: w315 -> [w414 w424]
                    tunnel: w314 -> [w413 _]
                    frame False {
                      n373 = local read "rightWaterOnFlag"() -> (w412:bool)
                      n374 = case shown="True" w412 {
                        tunnel: w416 -> [_ w421]
                        tunnel: [0 w421] -> w415
                        tunnel: w414 -> [_ w423]
                        tunnel: w413 -> [_ w422]
                        frame False {
                        }
                        frame True {
                          n375 = Add(x=w422, y=w421) -> (x+y=w420:u64)
                          n376 = Greater?(x=w423, y=w420) -> (0:w419:bool)
                          n377 = Not(x=w419) -> (.not. x?=w418:bool)
                          n378 = local write "rightWaterOnFlag"(w418) -> ()
                        }
                      }
                    }
                    frame True {
                      n379 = local write "manualWaterRight"(FALSE) -> ()
                      n380 = local write "rightWaterOnFlag"(TRUE) -> ()
                    }
                  }
                  n381 = shared-variable ".\\variables - network - RT (separate).lvlib\\stop - network"() -> (w409:bool)  [unwired: 1 in, 1 out]
                  n382 = local read "leftWaterOnFlag"() -> (w319:bool)
                  n383 = local read "rightWaterOnFlag"() -> (w313:bool)
                  n384 = local read "allowPunish"() -> (w309:bool)
                  n385 = local read "actuatorOn"() -> (w310:bool)
                  n386 = Select(t=states_def."exit", s=w409, f=w307) -> (s? t:f=w399:u32)
                  n387 = feedback-in #2(w399) -> ()
                  n388 = feedback-in #3(w399) -> ()
                  n389 = call "punish_check.vi"("input state"=w307, "lick"=w308, "allow punish"=w309) -> ("punish"=w306:bool)
                  n390 = Or(x=w319, y=w379) -> (x .or. y?=w378:bool)
                  n391 = Or(x=w313, y=w377) -> (x .or. y?=w376:bool)
                  n392 = Compound Arithmetic op=OR(w306, w310, w311) -> (w396:bool)
                  n393 = local read "ABORT"() -> (w343:bool)
                  n394 = Build Array(w380, w378, w376, w396) -> (w372:bool[])
                  n395 = Build Array (concatenate)(w375, w372, w374) -> (w373:bool[])
                  n396 = Boolean Array To Number(Boolean array=w373) -> (number=w325:u32)
                  n397 = Build Array (concatenate)(w366, w325, w323) -> (w364:dbl[])
                  n398 = Array Size(array=w364) -> (size(s)=w345:i32)
                  n399 = Build Array (concatenate)(w386, w364) -> (w384:dbl[])
                  n400 = local write "rtFIFOdataDim"(w345) -> ()
                  n401 = Array Size(array=w384) -> (size(s)=w381:i32)
                  n402 = Equal?(x=w381, y=w363) -> (x = y?=w383:bool)
                  n403 = Not Equal?(x=w345, y=9) -> (x != y?=w344:bool)
                  n404 = case shown="False" w383 {
                    tunnel: [w444 w451] -> w382
                    tunnel: w384 -> [w445 w448]
                    tunnel: [w445 sgl[] [] ("array type (2D Dbl)")] -> w385
                    tunnel: w359 -> [_ w447]
                    tunnel: w358 -> [w444 w446]
                    frame False {
                    }
                    frame True {
                      n405 = local read "rtFIFOtimeout"() -> (w449:u32)
                      n406 = RT FIFO Write(0:w447, 1:w448, 2:w449, 3:w446) -> (11:w451:errorcluster)  [unwired: 1 in, 3 out]
                    }
                  }
                  n407 = case shown="False" w344 {
                    frame False {
                    }
                    frame True {
                      n408 = One Button Dialog(message="The dimention of rtFIFOdata is not 4, pleae change the size of alocated network stream.") -> (true=w442:bool)  [unwired: 1 in]
                      n409 = local write "ABORT"(w442) -> ()
                    }
                  }
                  n410 = call-poly <vilib>:"DAQmx Write.vi"("task/channels in"=w348, "data"=w372, "error in"=w347) -> ("task out"=w403:refnum<k21>, "error out"=w402:errorcluster)  [unwired: 10 in, 1 out]
                  n411 = node-c288() -> ()  [unwired: 1 in, 1 out]
                }
                n412 = node-c288(5.0, 100 ("Priority")) -> (w231:T2)  [unwired: 1 in]
                n413 = timed-loop {
                  timing: w231 -> [_]
                  timing-out: [_] -> w230
                  tunnel: [w271] -> w208
                  tunnel: [w270] -> w207
                  tunnel: [w269] -> w210
                  tunnel: [w268] -> w209
                  tunnel: w229 -> [w267]
                  tunnel: w228 -> [w266]
                  tunnel: w215 -> [w265]
                  tunnel: w214 -> [w264]
                  shift-right: [w274] -> _
                  shift-left: w224 -> [w273]
                  stop <- w272 stop-if-true
                  n414 = node-c288() -> ()  [unwired: 1 in, 1 out]
                  n415 = property class="Network Stream Endpoint"(reference=w266, error in=w267) -> (reference out=w276:refnum<k21>, error out=w275:errorcluster, "Connected"=→"Is Connected":bool, "AvailElmntsForWrite"=→"Available Elements for Writing":i32)
                  n416 = RT FIFO Read(0:w265, 2:0, 3:w264) -> (8:w269:refnum<k33>, 9:w262:sgl[], 11:w268:errorcluster)  [unwired: 1 in, 2 out]
                  n417 = Empty Array?(array=w262) -> (empty?=w261:bool)
                  n418 = case shown="True" w261 {
                    tunnel: w262 -> [w284 _]
                    tunnel: [FALSE w289] -> w272
                    tunnel: w276 -> [w286 w287]
                    tunnel: w275 -> [w285 w288]
                    tunnel: [w279 w290] -> w274
                    tunnel: w273 -> [w282 w290]
                    tunnel: [w281 w287] -> w271
                    tunnel: [w280 w288] -> w270
                    frame False {
                      n419 = Increment(x=w282) -> (x+1=w279:i32)
                      n420 = shared-variable-write(w286, w285, w284) -> (w281:refnum<k21>, w280:errorcluster)  [unwired: 1 in, 1 out]
                      n421 = local write "stream counter"(w279) -> ()
                    }
                    frame True {
                      n422 = local read "ABORT"() -> (w289:bool)
                    }
                  }
                  n423 = node-c288() -> ()  [unwired: 1 in, 1 out]
                }
                n424 = node-c288(w230) -> (w198:errorcluster)
                n425 = node-c288(w234) -> (w200:errorcluster)
                n426 = Flush Stream(8:w207, 11:w208) -> (0:w206:errorcluster, 3:w205:refnum<k21>)  [unwired: 2 in, 1 out]
                n427 = RT FIFO Delete(0:w210, 3:w209) -> (11:w203:errorcluster)  [unwired: 1 in]
                n428 = Destroy Stream Endpoint(8:w206, 11:w205) -> (0:w204:errorcluster)
                n429 = node-c288(w232) -> (w199:errorcluster)
                n430 = stacked-sequence {
                  tunnel: w204 -> [w242]
                  tunnel: [w242] -> w197
                  frame #0 {
                    n431 = shared-variable "Sabrina-RT1\\variables - network - RT (separate).lvlib\\stop - network"(TRUE ("stop - network")) -> ()  [unwired: 1 in, 1 out]
                  }
                }
                n432 = Build Array(w195, w195, w195, w195) -> (w194:bool[])
                n433 = call-poly <vilib>:"DAQmx Write.vi"("task/channels in"=w202, "data"=w194, "error in"=w201) -> ("task out"=w175:refnum<k21>, "error out"=w174:errorcluster)  [unwired: 10 in, 1 out]
                n434 = call <vilib>:"DAQmx Stop Task.vi"("task/channels in"=w177, "error in"=w176) -> ("error out"=w173:errorcluster)  [unwired: 12 in, 1 out]
                n435 = call <vilib>:"DAQmx Stop Task.vi"("task/channels in"=w175, "error in"=w174) -> ("error out"=w172:errorcluster)  [unwired: 12 in, 1 out]
                n436 = Merge Errors(w192, w203) -> (w196:errorcluster)
                n437 = Merge Errors(w173, w172) -> (w178:errorcluster)
                n438 = Merge Errors(w200, w199, w198) -> (w179:errorcluster)
                n439 = Merge Errors(w179, w178, w196, w197) -> (w193:errorcluster)
                "error out" <- w193
                n440 = call <vilib>:"Simple Error Handler.vi"("error in (no error)"=w193) -> ()  [unwired: 4 in, 5 out]
              }
            }
          }
          frame #2 {
            n441 = Wait (ms)(milliseconds to wait=u32 100) -> ()  [unwired: 1 out]
          }
        }
      }
      n442 = UDP Close(connection ID=w23, 8:w22) -> (error out=w24:errorcluster)  [unwired: 1 out]
      n443 = UDP Close(connection ID=w18, 8:w19) -> (error out=w17:errorcluster)  [unwired: 1 out]
      n444 = call <vilib>:"Simple Error Handler.vi"("error in (no error)"=w24) -> ()  [unwired: 4 in, 5 out]
      n445 = call <vilib>:"Simple Error Handler.vi"("error in (no error)"=w17) -> ()  [unwired: 4 in, 5 out]
    }
  }
